vi "start.vi"(8 "error in (no error)":errorcluster, 11 "DL090202FPGAClock in":refnum<class "ClockDL090202FPGA.lvclass">) -> (0 "error out":errorcluster, 3 "DL090202FPGAClock out":refnum<class "ClockDL090202FPGA.lvclass">)   [LabVIEW 2010, in "ClockDL090202FPGA.lvclass"]
uses:
  ClockDL090202FPGA.lvclass
  ClockDL090202FPGA.lvclass/ClockDL090202FPGA.ctl
  FPGAWrapper/GenericFPGAWrapper/GenericFPGAWrapper/GenericFPGAWrapper.lvclass
  common/classes/ErrorController/ErrorController/class_data.vi
  common/classes/ErrorController/ErrorController/ErrorController.lvclass
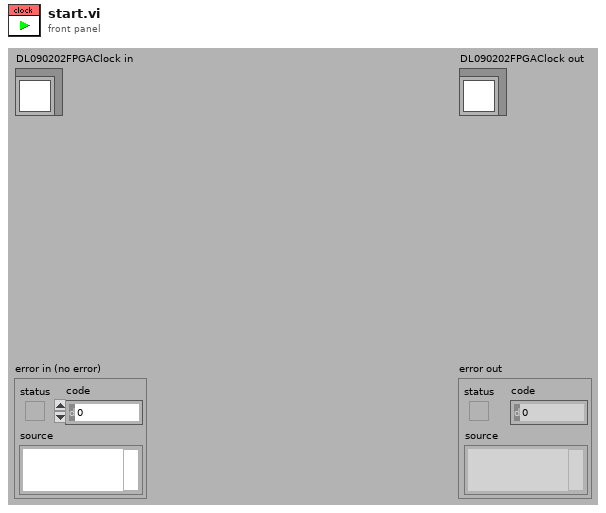
[diagram p1: front panel]
types:
  T1 = typedef "ClockDL090202FPGA.lvclass/type_enum.ctl" = enum16{"pixel clock", "gate 1", "gate 2", "gate 3"}
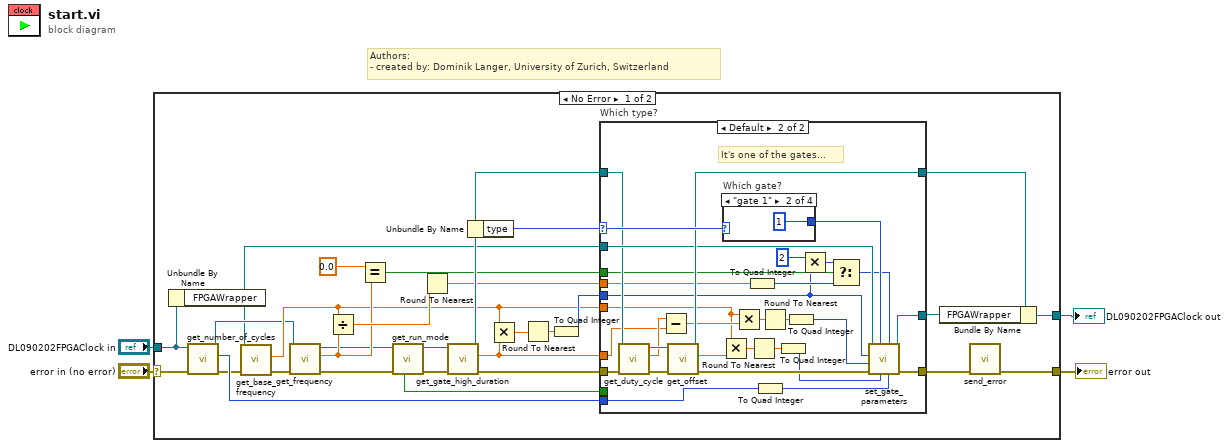
[diagram p0: block diagram]
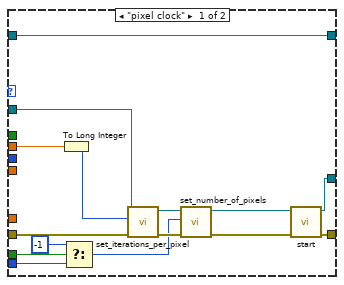
[diagram p2: hidden frame]
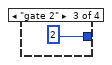
[diagram p4: hidden frame]
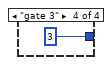
[diagram p5: hidden frame]
diagram:
  # "Authors: \n- created by: Dominik Langer, University of Zurich, Switzerland"
  n1 = case shown="No Error" "error in (no error)" {
    selector: "error in (no error)" -> [w25 w85]
    tunnel: [w6 w85] -> w3
    tunnel: [w26 w84] -> w1
    tunnel: "DL090202FPGAClock in" -> [w12 w84]
    frame No Error {
      n2 = Unbundle By Name(w12) -> ("FPGAWrapper"=w7:refnum<class "GenericFPGAWrapper.lvclass">)
      n3 = call-dynamic "get_number_of_cycles.vi"("error in (no error)"=w25, "GenericClock.lvclass in"=w12) -> ("error out"=w11:errorcluster, "number of cycles"=w22:i32, "GenericClock.lvclass out"=w8:refnum<class "ClockDL090202FPGA.lvclass">)  [unwired: 7 out]
      n4 = call-dynamic "get_base_frequency.vi"("error in (no error)"=w11, "GenericFPGAWrapper in"=w7) -> ("error out"=w9:errorcluster, "base frequency"=w10:dbl[unit])  [unwired: 7 in, 1 out]
      n5 = call-dynamic "get_frequency.vi"("error in (no error)"=w9, "GenericClock.lvclass in"=w8) -> ("error out"=w17:errorcluster, "frequency"=w19:dbl[unit], "GenericClock.lvclass out"=w15:refnum<class "ClockDL090202FPGA.lvclass">)  [unwired: 7 out]
      n6 = Divide(x=w10, y=w19) -> (x/y=w21:dbl)
      n7 = Equal?(x=dbl[unit] 0.0, y=w19) -> (x = y?=w18:bool)
      n8 = call-dynamic "get_run_mode.vi"("error in (no error)"=w17, "GenericPlugin in"=w15) -> ("error out"=w16:errorcluster, "GenericPlugin out"=w14:refnum<class "ClockDL090202FPGA.lvclass">, "is free run?"=w13:bool)  [unwired: 5 in, 2 out]
      n9 = Round To Nearest(number=w21) -> (nearest integer value=w23:dbl)
      n10 = call-dynamic "get_gate_high_duration.vi"("error in (no error)"=w16, "GenericClock.lvclass in"=w14) -> ("error out"=w32:errorcluster, "gate high duration"=w24:dbl[unit], "GenericClock.lvclass out"=w28:refnum<class "ClockDL090202FPGA.lvclass">)  [unwired: 7 out]
      n11 = Unbundle By Name(w28) -> ("type"=w33:T1)
      n12 = Multiply(x=w10, y=w24) -> (x*y=w29:dbl)
      n13 = Round To Nearest(number=w29) -> (nearest integer value=w31:dbl)
      n14 = To Quad Integer(1:w31) -> (0:w30:i64)
      n15 = case "Which type?" shown="Default" w33 {
        selector: w33 -> [_ w78]
        tunnel: w23 -> [w42 w56]
        tunnel: w7 -> [w49 w72]
        tunnel: w32 -> [w47 w69]
        tunnel: w22 -> [w39 w58]
        tunnel: [w46 w80] -> w5
        tunnel: [w45 w79] -> w34
        tunnel: w28 -> [w44 w67]
        tunnel: [w44 w75] -> w27
        tunnel: w30 -> [_ w51]
        tunnel: w10 -> [_ w62]
        tunnel: w24 -> [_ w64]
        tunnel: w18 -> [_ w55]
        tunnel: w13 -> [w40 _]
        frame "pixel clock" {
          n16 = To Long Integer(number=w42) -> (32bit integer=w41:i32)
          n17 = Select(t=-1, s=w40, f=w39) -> (s? t:f=w37:i32)
          n18 = call-dynamic "set_iterations_per_pixel.vi"("error in (no error)"=w47, "iterations per pixel"=w41, "GenericFPGAWrapper in"=w49) -> ("error out"=w48:errorcluster, "GenericFPGAWrapper out"=w36:refnum<class "GenericFPGAWrapper.lvclass">)  [unwired: 7 out]
          n19 = call-dynamic "set_number_of_pixels.vi"("error in (no error)"=w48, "number of pixels"=w37, "GenericFPGAWrapper in"=w36) -> ("error out"=w43:errorcluster, "GenericFPGAWrapper out"=w35:refnum<class "GenericFPGAWrapper.lvclass">)  [unwired: 7 out]
          n20 = call-dynamic "start.vi"("error in (no error)"=w43, "GenericFPGAWrapper in"=w35) -> ("error out"=w46:errorcluster, "GenericFPGAWrapper out"=w45:refnum<class "GenericFPGAWrapper.lvclass">)  [unwired: 8 out]
        }
        frame Default {
          # "It's one of the gates..."
          n21 = call-dynamic "get_duty_cycle.vi"("error in (no error)"=w69, "GenericClock.lvclass in"=w67) -> ("error out"=w68:errorcluster, "duty cycle"=w65:dbl[unit], "GenericClock.lvclass out"=w66:refnum<class "ClockDL090202FPGA.lvclass">)  [unwired: 7 out]
          n22 = Subtract(x=w65, y=w64) -> (x-y=w63:dbl[unit])
          n23 = call-dynamic "get_offset.vi"("error in (no error)"=w68, "GenericClock.lvclass in"=w66) -> ("error out"=w76:errorcluster, "offset"=w74:dbl[unit], "GenericClock.lvclass out"=w75:refnum<class "ClockDL090202FPGA.lvclass">)  [unwired: 7 out]
          n24 = Multiply(x=w62, y=w74) -> (x*y=w71:dbl)
          n25 = case "Which gate?" shown="\"gate 1\"" w78 {
            tunnel: [_ 1 2 3] -> w77
            frame Default {
            }
            frame "gate 1" {
            }
            frame "gate 2" {
            }
            frame "gate 3" {
            }
          }
          n26 = Multiply(x=w62, y=w63) -> (x*y=w61:dbl)
          n27 = To Quad Integer(1:w56) -> (0:w54:i64)
          n28 = Round To Nearest(number=w71) -> (nearest integer value=w73:dbl)
          n29 = To Quad Integer(1:w58) -> (0:w57:i64)
          n30 = Round To Nearest(number=w61) -> (nearest integer value=w60:dbl)
          n31 = To Quad Integer(1:w73) -> (0:w70:i64)
          n32 = To Quad Integer(1:w60) -> (0:w59:i64)
          n33 = Multiply(x=i64 2, y=w51) -> (x*y=w52:i64)
          n34 = Select(t=w52, s=w55, f=w54) -> (s? t:f=w53:i64)
          n35 = call-dynamic "set_gate_parameters.vi"("repetitions"=w57, "pulse duration (iterations)"=w53, "offset duration (iterations)"=w70, "clock index"=w77, "error in (no error)"=w76, "low phase duration (iterations)"=w59, "high phase duration (iterations)"=w51, "GenericFPGAWrapper in"=w72) -> ("error out"=w80:errorcluster, "GenericFPGAWrapper out"=w79:refnum<class "GenericFPGAWrapper.lvclass">)  [unwired: 2 out]
        }
      }
      n36 = Bundle By Name(cluster=w27, "FPGAWrapper"=w34) -> (w26:refnum<class "ClockDL090202FPGA.lvclass">)
      n37 = call "send_error.vi"("error in (no error)"=w5) -> ("error out"=w6:errorcluster)  [unwired: 10 in]
    }
    frame Error {
    }
  }
  "error out" <- w3
  "DL090202FPGAClock out" <- w1
